vi "onBoard LED all test.vi"() -> ()   [LabVIEW 2019]
panel:
  in  "LED[3:0]":u8=5 format="%.0b"
  out "Error Out":errorcluster
  in  "error in":errorcluster
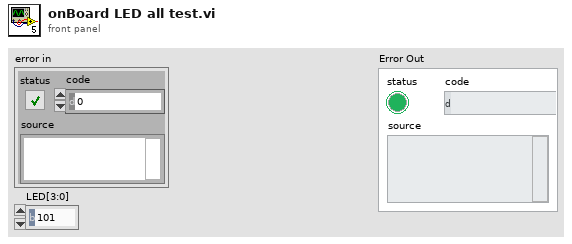
[diagram p1: front panel]
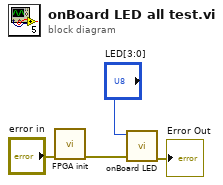
[diagram p0: block diagram]
diagram:
  n1 = call "FPGA init.vi"("error in"="error in") -> ("error out"=w3:errorcluster)  [unwired: 9 in, 1 out]
  n2 = call "onBoard LED.vi"("Error In"=w3, "LED[3:0]"="LED[3:0]") -> ("Error Out"=→"Error Out":errorcluster)  [unwired: 9 in]
